vi "Execute Network Operation.vi"(7 "Operation":T1, 8 "error in (no error)":errorcluster, 10 "Message":string, 11 "Listener In.lvclass":refnum<class "Listener.lvclass">) -> (0 "error out":errorcluster, 3 "Listener Out.lvclass":refnum<class "Listener.lvclass">)   [LabVIEW 2019, in "Listener.lvclass"]
doc: "Reads/Writes data using the specified protocol.\nInput: \nListener Object\nMessage: The \"packet\" which will be sent through the selected protocol\nOpeartion: Read/Write operation on the specified protocol"
uses:
  Listener.lvclass
  ListenerClassControls/Operation.ctl
  Constants.vi
  <vilib>/Utility/error.llb/Error Cluster From Error Code.vi
  Protocols.lvlib
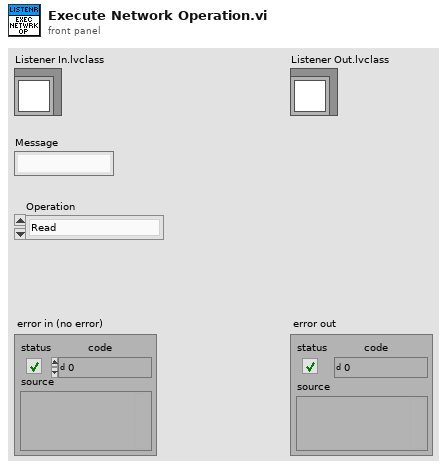
[diagram p1: front panel]
types:
  T1 = typedef "Listener.lvclass/Operation.ctl" = enum16{"Read", "Write"}
  T2 = enum16{"Standard", "Buffered", "CRLF", "Immediate"}
  T3 = typedef "Listener.lvclass/Protocol.ctl" = enum16{"RS-XXX", "AK RS-XXX", "VISA", "TCPIP", "AK TCPIP", "UDP", "GPIB ConvBox"}
  T4 = typedef "Listener.lvclass/UDP Data Structure.ctl" = cluster{"UDP connection ID":refnum<k16>, "Local Address":string, "Local Port":u16, "Target IP Address":string, "Target Port":u16, "Data":string}
  T5 = typedef "Listener.lvclass/TCP Data Structure.ctl" = cluster{"TCP|IP connection ID":refnum<k5>, "IP Address":string, "Port":u16, "Data":string}
  T6 = typedef "Listener.lvclass/AK TCP Data Structure.ctl" = cluster{"TCP|IP connection ID":refnum<k5>, "IP Address":string, "Port":u16, "Data":string, "Current Command Code":string}
  T7 = typedef "Listener.lvclass/VISA Data Structure.ctl" = cluster{"Protocol Ref Out":refnum<visa-resource-name>, "Listener Ref Out":refnum<visa-resource-name>, "Data Length":u32, "Data":string}
  T8 = typedef "Listener.lvclass/RS-xxx Data Structure.ctl" = cluster{"Protocol Port Ref":refnum<visa-resource-name>, "Listener Port Ref":refnum<visa-resource-name>, "Virtual COM Port Settings 1":cluster{"Port":string, "Baud Rate":u32, "Data Bits":u16, "Parity":enum16{"None", "Odd", "Even", "Mark", "Space"}, "Stop Bits":u16, "Flow Control":u16, "XON":enum16{"NUL", "SOH", "STX", "ETX", "EOT", "ENQ", "ACK", "BEL", "BS", "HT", "LF", "VT", "FF", "CR", "SO", "SI", "DLE", "DC1", "DC2", "DC3", "DC4", "NAK", "SYN", "ETB", "CAN", "EM", "SUB", "ESC", "FS", "GS", "RS", "US", "SP", "!", "\"", "#", "$", "%", "&", "'", "(", ")", "*", "+", ",", "- (-)", ".", "/", "0", "1", "2", "3", "4", "5", "6", "7", "8", "9", ":", ";", "<", "=", ">", "?", "@", "A", "B", "C", "D", "E", "F", "G", "H", "I", "J", "K", "L", "M", "N", "O", "P", "Q", "R", "S", "T", "U", "V", "W", "X", "Y", "Z", "[", "\\", "]", "^", "_", "`", "a", "b", "c", "d", "e", "f", "g", "h", "i", "j", "k", "l", "m", "n", "o", "p", "q", "r", "s", "t", "u", "v", "w", "x", "y", "z", "{", "|", "}", "~"}, "XOFF":enum16{"NUL", "SOH", "STX", "ETX", "EOT", "ENQ", "ACK", "BEL", "BS", "HT", "LF", "VT", "FF", "CR", "SO", "SI", "DLE", "DC1", "DC2", "DC3", "DC4", "NAK", "SYN", "ETB", "CAN", "EM", "SUB", "ESC", "FS", "GS", "RS", "US", "SP", "!", "\"", "#", "$", "%", "&", "'", "(", ")", "*", "+", ",", "- (-)", ".", "/", "0", "1", "2", "3", "4", "5", "6", "7", "8", "9", ":", ";", "<", "=", ">", "?", "@", "A", "B", "C", "D", "E", "F", "G", "H", "I", "J", "K", "L", "M", "N", "O", "P", "Q", "R", "S", "T", "U", "V", "W", "X", "Y", "Z", "[", "\\", "]", "^", "_", "`", "a", "b", "c", "d", "e", "f", "g", "h", "i", "j", "k", "l", "m", "n", "o", "p", "q", "r", "s", "t", "u", "v", "w", "x", "y", "z", "{", "|", "}", "~"}, "End Read on Termination Character":bool, "End Write on Termination Character":bool, "Termination Character":u8}, "Virtual COM Port Settings 2":cluster{"Port":string, "Baud Rate":u32, "Data Bits":u16, "Parity":enum16{"None", "Odd", "Even", "Mark", "Space"}, "Stop Bits":u16, "Flow Control":u16, "XON":enum16{"NUL", "SOH", "STX", "ETX", "EOT", "ENQ", "ACK", "BEL", "BS", "HT", "LF", "VT", "FF", "CR", "SO", "SI", "DLE", "DC1", "DC2", "DC3", "DC4", "NAK", "SYN", "ETB", "CAN", "EM", "SUB", "ESC", "FS", "GS", "RS", "US", "SP", "!", "\"", "#", "$", "%", "&", "'", "(", ")", "*", "+", ",", "- (-)", ".", "/", "0", "1", "2", "3", "4", "5", "6", "7", "8", "9", ":", ";", "<", "=", ">", "?", "@", "A", "B", "C", "D", "E", "F", "G", "H", "I", "J", "K", "L", "M", "N", "O", "P", "Q", "R", "S", "T", "U", "V", "W", "X", "Y", "Z", "[", "\\", "]", "^", "_", "`", "a", "b", "c", "d", "e", "f", "g", "h", "i", "j", "k", "l", "m", "n", "o", "p", "q", "r", "s", "t", "u", "v", "w", "x", "y", "z", "{", "|", "}", "~"}, "XOFF":enum16{"NUL", "SOH", "STX", "ETX", "EOT", "ENQ", "ACK", "BEL", "BS", "HT", "LF", "VT", "FF", "CR", "SO", "SI", "DLE", "DC1", "DC2", "DC3", "DC4", "NAK", "SYN", "ETB", "CAN", "EM", "SUB", "ESC", "FS", "GS", "RS", "US", "SP", "!", "\"", "#", "$", "%", "&", "'", "(", ")", "*", "+", ",", "- (-)", ".", "/", "0", "1", "2", "3", "4", "5", "6", "7", "8", "9", ":", ";", "<", "=", ">", "?", "@", "A", "B", "C", "D", "E", "F", "G", "H", "I", "J", "K", "L", "M", "N", "O", "P", "Q", "R", "S", "T", "U", "V", "W", "X", "Y", "Z", "[", "\\", "]", "^", "_", "`", "a", "b", "c", "d", "e", "f", "g", "h", "i", "j", "k", "l", "m", "n", "o", "p", "q", "r", "s", "t", "u", "v", "w", "x", "y", "z", "{", "|", "}", "~"}, "End Read on Termination Character":bool, "End Write on Termination Character":bool, "Termination Character":u8}, "Data":string, "Data Length":u32}
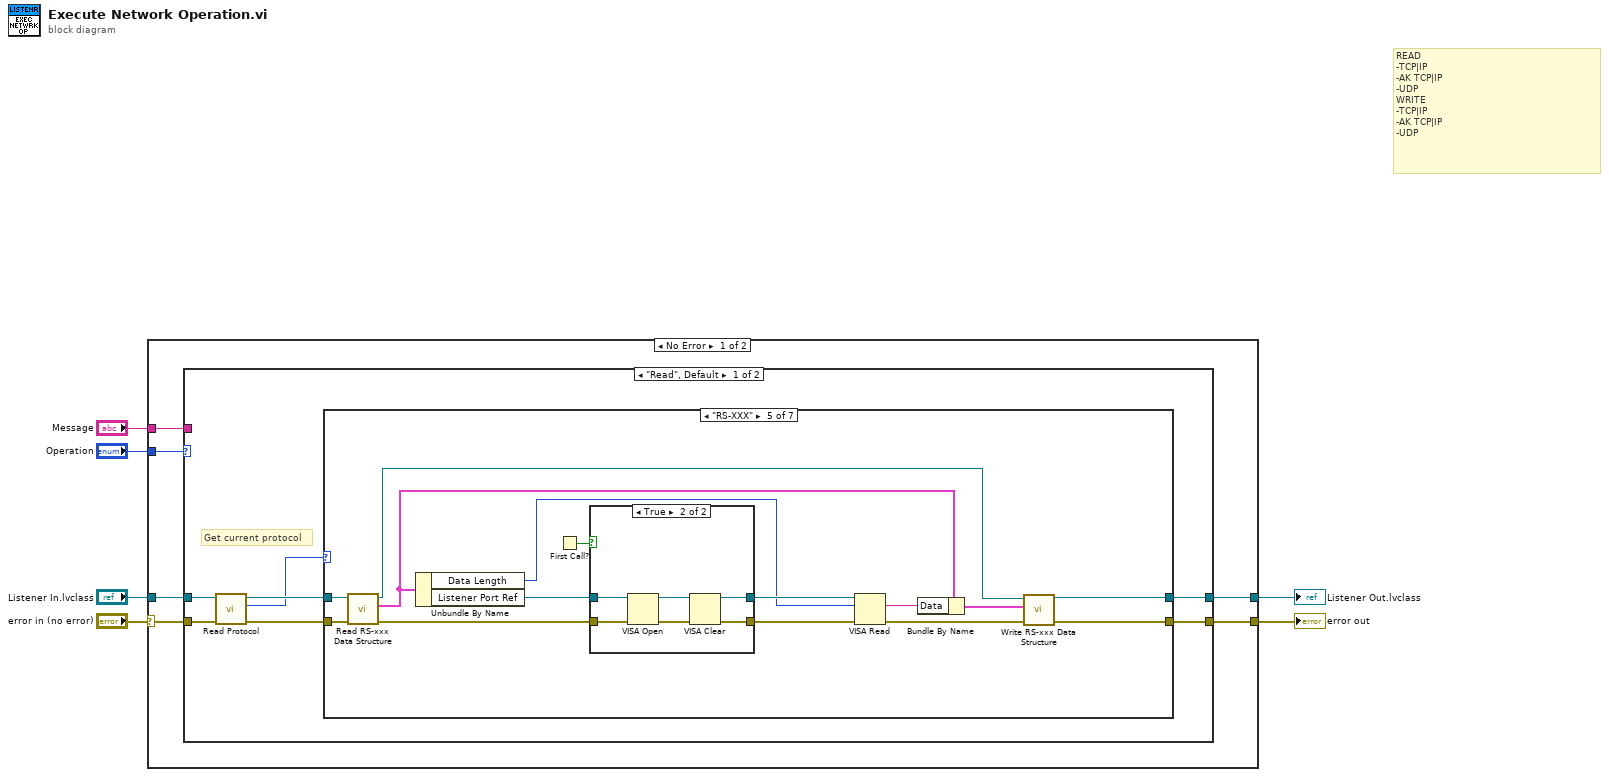
[diagram p0: block diagram]
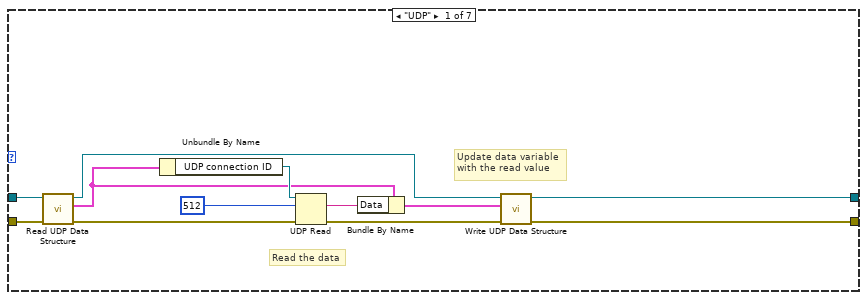
[diagram p2: hidden frame]
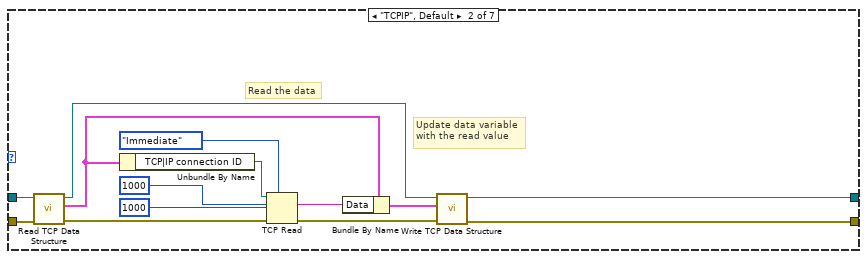
[diagram p3: hidden frame]
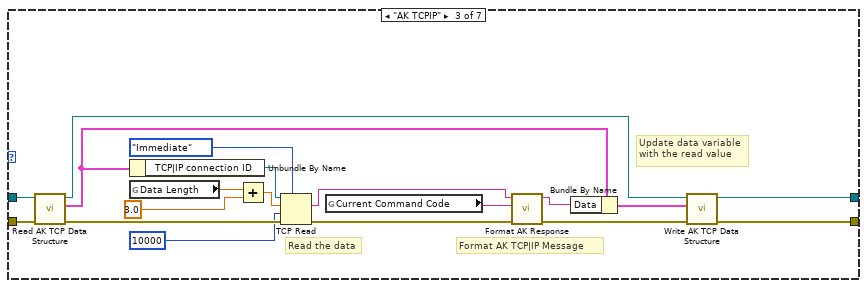
[diagram p4: hidden frame]
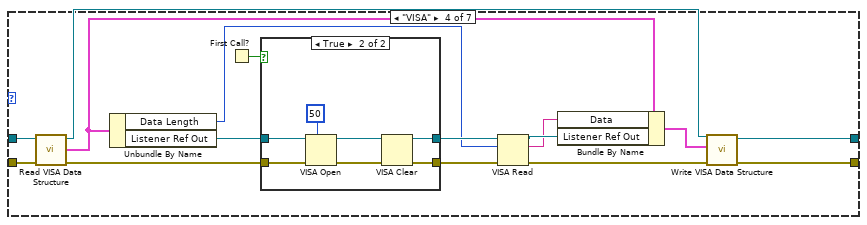
[diagram p5: hidden frame]
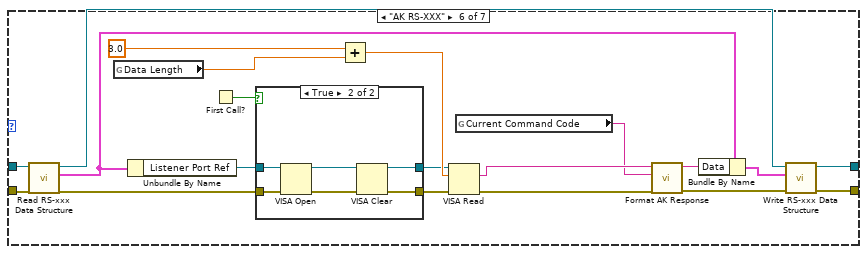
[diagram p8: hidden frame]
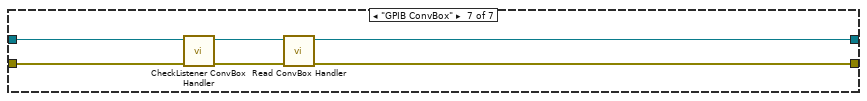
[diagram p10: hidden frame]
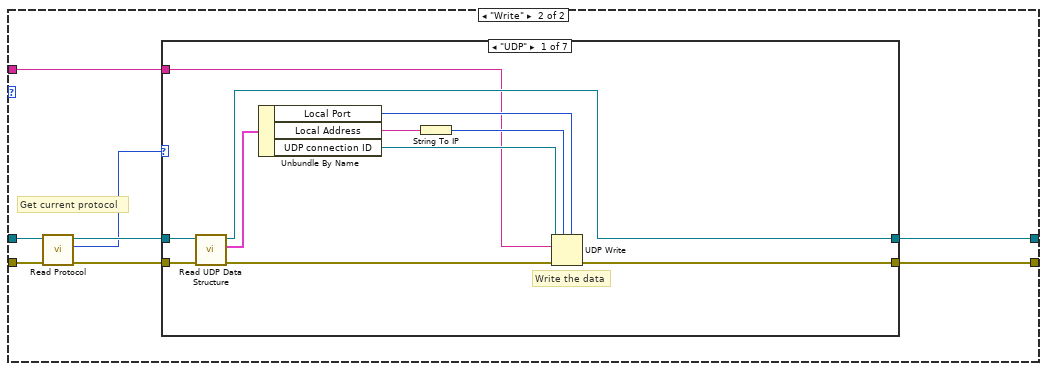
[diagram p11: hidden frame]
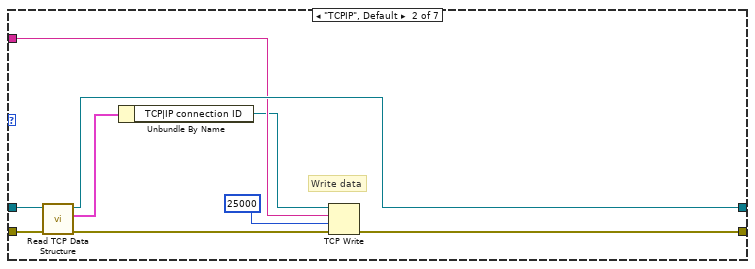
[diagram p12: hidden frame]
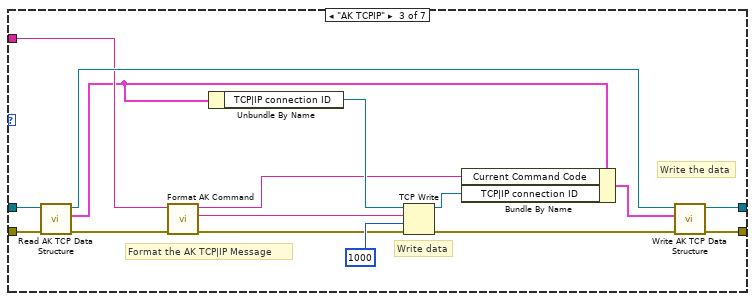
[diagram p13: hidden frame]
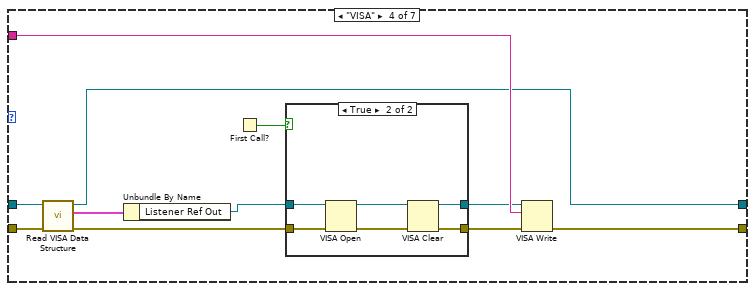
[diagram p14: hidden frame]
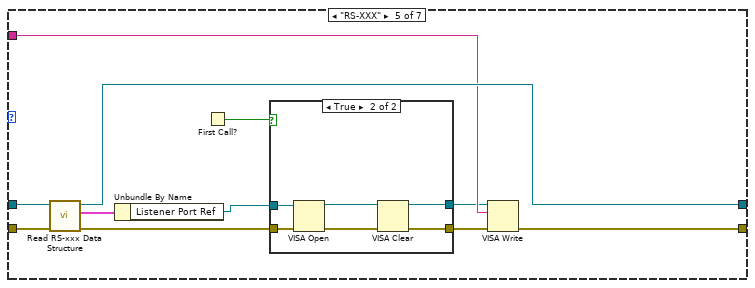
[diagram p16: hidden frame]
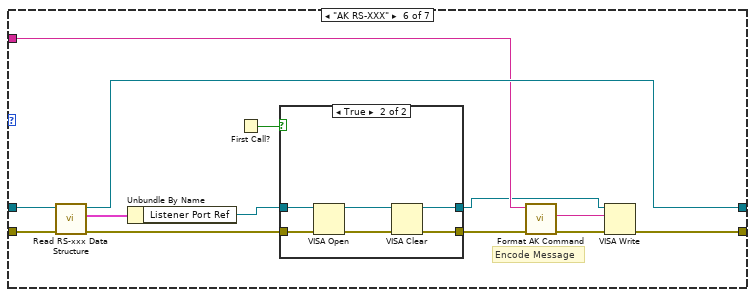
[diagram p18: hidden frame]
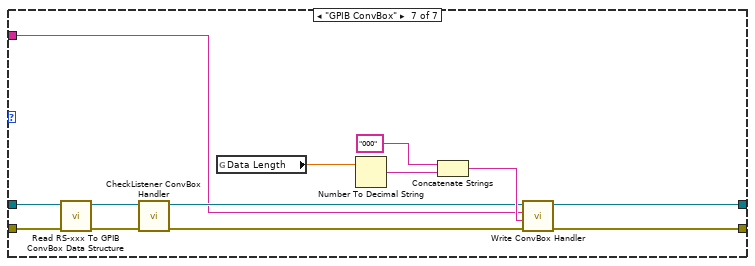
[diagram p20: hidden frame]
diagram:
  # "READ\n-TCP|IP\n-AK TCP|IP\n-UDP\nWRITE\n-TCP|IP\n-AK TCP|IP\n-UDP"
  n1 = case shown="No Error" "error in (no error)" {
    selector: "error in (no error)" -> [w9 w263]
    tunnel: "Listener In.lvclass" -> [w12 w264]
    tunnel: [w11 w263] -> w5
    tunnel: [w10 w264] -> w4
    tunnel: "Operation" -> [w8 _]
    tunnel: "Message" -> [w7 _]
    frame No Error {
      n2 = case shown="\"Read\", Default" w8 {
        tunnel: w9 -> [w19 w152]
        tunnel: w12 -> [w18 w149]
        tunnel: [w15 w153] -> w11
        tunnel: [w14 w154] -> w10
        tunnel: w7 -> [_ w147]
        frame "Read", Default {
          # "Get current protocol"
          n3 = call-dynamic "Read Protocol.vi"("error in (no error)"=w19, "Listener in"=w18) -> ("error out"=w17:errorcluster, "Protocol"=w13:T3, "Listener out"=w16:refnum<class "Listener.lvclass">)  [unwired: 7 in]
          n4 = case shown="\"RS-XXX\"" w13 {
            tunnel: w17 -> [w31 w45 w52 w79 w103 w130 w142]
            tunnel: w16 -> [w30 w44 w53 w80 w104 w129 w144]
            tunnel: [w28 w42 w50 w74 w97 w128 w145] -> w14
            tunnel: [w29 w43 w51 w77 w96 w113 w146] -> w15
            frame "UDP" {
              # "Read the data"
              # "Update data variable\nwith the read value"
              n5 = call-dynamic "Read UDP Data Structure.vi"("error in (no error)"=w31, "Listener in"=w30) -> ("error out"=w27:errorcluster, "UDP Data Structure"=w24:T4, "Listener out"=w21:refnum<class "Listener.lvclass">)  [unwired: 7 in]
              n6 = Unbundle By Name(w24) -> ("UDP connection ID"=w25:refnum<k16>)
              n7 = UDP Read(connection ID=w25, max size (548)=512, 8:w27) -> (data out=w23:string, error out=w22:errorcluster)  [unwired: 1 in, 3 out]
              n8 = Bundle By Name(cluster=w24, "Data"=w23) -> (w20:T4)
              n9 = call-dynamic "Write UDP Data Structure.vi"("error in (no error)"=w22, "UDP Data Structure"=w20, "Listener in"=w21) -> ("error out"=w29:errorcluster, "Listener out"=w28:refnum<class "Listener.lvclass">)  [unwired: 7 in]
            }
            frame "TCPIP", Default {
              # "Update data variable\nwith the read value"
              # "Read the data"
              n10 = call-dynamic "Read TCP Data Structure.vi"("error in (no error)"=w45, "Listener in"=w44) -> ("error out"=w40:errorcluster, "TCP|IP Data Structure"=w39:T5, "Listener out"=w35:refnum<class "Listener.lvclass">)  [unwired: 7 in]
              n11 = Unbundle By Name(w39) -> ("TCP|IP connection ID"=w34:refnum<k5>)
              n12 = TCP Read(connection ID=w34, bytes to read=1000, error in (no error)=w40, 7:T2."Immediate" ("mode (standard)"), 9:1000 ("timeout ms (25000)")) -> (data out=w38:string, error out=w36:errorcluster)  [unwired: 1 out]
              n13 = Bundle By Name(cluster=w39, "Data"=w38) -> (w37:T5)
              n14 = call-dynamic "Write TCP Data Structure.vi"("error in (no error)"=w36, "TCP|IP Data Structure"=w37, "Listener in"=w35) -> ("error out"=w43:errorcluster, "Listener out"=w42:refnum<class "Listener.lvclass">)  [unwired: 7 in]
            }
            frame "AK TCPIP" {
              # "Format AK TCP|IP Message"
              # "Update data variable\nwith the read value"
              # "Read the data"
              n15 = call-dynamic "Read AK TCP Data Structure.vi"("error in (no error)"=w52, "Listener in"=w53) -> ("error out"=w63:errorcluster, "TCP|IP Data Structure"=w60:T6, "Listener out"=w56:refnum<class "Listener.lvclass">)  [unwired: 7 in]
              n16 = Unbundle By Name(w60) -> ("TCP|IP connection ID"=w64:refnum<k5>)
              n17 = global read "Constants.vi" "Data Length"() -> (w49:dbl)
              n18 = Add(x=w49, y=3.0) -> (x+y=w47:dbl)
              n19 = TCP Read(connection ID=w64, bytes to read=w47, error in (no error)=w63, 7:T2."Immediate" ("mode (standard)"), 9:10000 ("timeout ms (25000)")) -> (data out=w61:string, error out=w62:errorcluster)  [unwired: 1 out]
              n20 = global read "Constants.vi" "Current Command Code"() -> (w46:string)
              n21 = call "Format AK Response.vi"("error in (no error)"=w62, "Current Command Code"=w46, "Response"=w61) -> ("error out"=w58:errorcluster, "Data"=w59:string)  [unwired: 7 in]
              n22 = Bundle By Name(cluster=w60, "Data"=w59) -> (w57:T6)
              n23 = call-dynamic "Write AK TCP Data Structure.vi"("error in (no error)"=w58, "TCP|IP Data Structure"=w57, "Listener in"=w56) -> ("error out"=w51:errorcluster, "Listener out"=w50:refnum<class "Listener.lvclass">)  [unwired: 7 in]
            }
            frame "VISA" {
              n24 = call-dynamic "Read VISA Data Structure.vi"("error in (no error)"=w79, "Listener in"=w80) -> ("error out"=w71:errorcluster, "VISA Data Structure"=w78:T7, "Listener out"=w75:refnum<class "Listener.lvclass">)  [unwired: 7 in]
              n25 = Unbundle By Name(w78) -> ("Data Length"=w68:u32, "Listener Ref Out"=w67:refnum<visa-resource-name>)
              n26 = First Call?() -> (First Call?: T/F=w72:bool)
              n27 = case shown="True" w72 {
                tunnel: w67 -> [w82 w89]
                tunnel: w71 -> [w81 w88]
                tunnel: [w81 w87] -> w70
                tunnel: [w82 w86] -> w69
                frame False {
                }
                frame True {
                  n28 = VISA Open(timeout (0)=u32 50 ("VISA Open timeout (0)"), error in (no error)=w88, VISA resource name=w89) -> (VISA resource name=w84:refnum<visa-resource-name>, error out=w85:errorcluster)  [unwired: 2 in]
                  n29 = VISA Clear(VISA resource name=w84, error in (no error)=w85) -> (VISA resource name out=w86:refnum<visa-resource-name>, error out=w87:errorcluster)
                }
              }
              n30 = VISA Read(VISA resource name=w69, byte count=w68, error in (no error)=w70) -> (VISA resource name out=w66:refnum<visa-resource-name>, read buffer=w65:string, error out=w73:errorcluster)  [unwired: 1 out]
              n31 = Bundle By Name(cluster=w78, "Data"=w65, "Listener Ref Out"=w66) -> (w76:T7)
              n32 = call-dynamic "Write VISA Data Structure.vi"("error in (no error)"=w73, "VISA Data Structure"=w76, "Listener in"=w75) -> ("error out"=w77:errorcluster, "Listener out"=w74:refnum<class "Listener.lvclass">)  [unwired: 7 in]
            }
            frame "RS-XXX" {
              n33 = call-dynamic "Read RS-xxx Data Structure.vi"("error in (no error)"=w103, "Listener in"=w104) -> ("error out"=w93:errorcluster, "RS-xxx Data Structure"=w102:T8, "Listener out"=w99:refnum<class "Listener.lvclass">)  [unwired: 7 in]
              n34 = Unbundle By Name(w102) -> ("Data Length"=w90:u32, "Listener Port Ref"=w94:refnum<visa-resource-name>)
              n35 = First Call?() -> (First Call?: T/F=w95:bool)
              n36 = case shown="True" w95 {
                tunnel: w94 -> [w106 w112]
                tunnel: w93 -> [w105 w110]
                tunnel: [w105 w108] -> w92
                tunnel: [w106 w107] -> w91
                frame False {
                }
                frame True {
                  n37 = VISA Open(error in (no error)=w110, VISA resource name=w112) -> (VISA resource name=w111:refnum<visa-resource-name>, error out=w109:errorcluster)  [unwired: 3 in]
                  n38 = VISA Clear(VISA resource name=w111, error in (no error)=w109) -> (VISA resource name out=w107:refnum<visa-resource-name>, error out=w108:errorcluster)
                }
              }
              n39 = VISA Read(VISA resource name=w91, byte count=w90, error in (no error)=w92) -> (read buffer=w101:string, error out=w98:errorcluster)  [unwired: 2 out]
              n40 = Bundle By Name(cluster=w102, "Data"=w101) -> (w100:T8)
              n41 = call-dynamic "Write RS-xxx Data Structure.vi"("error in (no error)"=w98, "RS-xxx Data Structure"=w100, "Listener in"=w99) -> ("error out"=w96:errorcluster, "Listener out"=w97:refnum<class "Listener.lvclass">)  [unwired: 7 in]
            }
            frame "AK RS-XXX" {
              n42 = call-dynamic "Read RS-xxx Data Structure.vi"("error in (no error)"=w130, "Listener in"=w129) -> ("error out"=w117:errorcluster, "RS-xxx Data Structure"=w131:T8, "Listener out"=w132:refnum<class "Listener.lvclass">)  [unwired: 7 in]
              n43 = global read "Constants.vi" "Data Length"() -> (w124:dbl)
              n44 = Unbundle By Name(w131) -> ("Listener Port Ref"=w116:refnum<visa-resource-name>)
              n45 = First Call?() -> (First Call?: T/F=w118:bool)
              n46 = case shown="True" w118 {
                tunnel: w116 -> [w134 w140]
                tunnel: w117 -> [w133 w139]
                tunnel: [w133 w137] -> w114
                tunnel: [w134 w136] -> w115
                frame False {
                }
                frame True {
                  n47 = VISA Open(error in (no error)=w139, VISA resource name=w140) -> (VISA resource name=w135:refnum<visa-resource-name>, error out=w138:errorcluster)  [unwired: 3 in]
                  n48 = VISA Clear(VISA resource name=w135, error in (no error)=w138) -> (VISA resource name out=w136:refnum<visa-resource-name>, error out=w137:errorcluster)
                }
              }
              n49 = Add(x=3.0 ("y"), y=w124) -> (x+y=w125:dbl)
              n50 = VISA Read(VISA resource name=w115, byte count=w125, error in (no error)=w114) -> (read buffer=w122:string, error out=w120:errorcluster)  [unwired: 2 out]
              n51 = global read "Constants.vi" "Current Command Code"() -> (w121:string)
              n52 = call "Format AK Response.vi"("error in (no error)"=w120, "Current Command Code"=w121, "Response"=w122) -> ("error out"=w119:errorcluster, "Data"=w127:string)  [unwired: 7 in]
              n53 = Bundle By Name(cluster=w131, "Data"=w127) -> (w126:T8)
              n54 = call-dynamic "Write RS-xxx Data Structure.vi"("error in (no error)"=w119, "RS-xxx Data Structure"=w126, "Listener in"=w132) -> ("error out"=w113:errorcluster, "Listener out"=w128:refnum<class "Listener.lvclass">)  [unwired: 7 in]
            }
            frame "GPIB ConvBox" {
              n55 = call "CheckListener ConvBox Handler.vi"("error in (no error)"=w142, "Listener in"=w144) -> ("error out"=w141:errorcluster, "Listener out"=w143:refnum<class "Listener.lvclass">)  [unwired: 8 in]
              n56 = call "Read ConvBox Handler.vi"("error in (no error)"=w141, "Listener in"=w143) -> ("error out"=w146:errorcluster, "Listener out"=w145:refnum<class "Listener.lvclass">)  [unwired: 8 in]
            }
          }
        }
        frame "Write" {
          # "Get current protocol"
          n57 = call-dynamic "Read Protocol.vi"("error in (no error)"=w152, "Listener in"=w149) -> ("error out"=w151:errorcluster, "Protocol"=w148:T3, "Listener out"=w150:refnum<class "Listener.lvclass">)  [unwired: 7 in]
          n58 = case shown="\"UDP\"" w148 {
            tunnel: [w162 w174 w178 w197 w216 w238 w262] -> w154
            tunnel: [w163 w173 w177 w196 w219 w239 w261] -> w153
            tunnel: w150 -> [w164 w171 w176 w201 w217 w241 w255]
            tunnel: w151 -> [w165 w172 w179 w200 w218 w240 w254]
            tunnel: w147 -> [w155 w170 w180 w199 w215 w235 w250]
            frame "UDP" {
              # "Write the data"
              n59 = call-dynamic "Read UDP Data Structure.vi"("error in (no error)"=w165, "Listener in"=w164) -> ("error out"=w159:errorcluster, "UDP Data Structure"=w161:T4, "Listener out"=w162:refnum<class "Listener.lvclass">)  [unwired: 7 in]
              n60 = Unbundle By Name(w161) -> ("Local Port"=w158:u16, "Local Address"=w157:string, "UDP connection ID"=w160:refnum<k16>)
              n61 = String To IP(1:w157) -> (0:w156:u32)
              n62 = UDP Write(address=w156, port or service name=w158, connection ID=w160, data in=w155, 8:w159) -> (error out=w163:errorcluster)  [unwired: 1 in, 1 out]
            }
            frame "TCPIP", Default {
              # "Write data"
              n63 = call-dynamic "Read TCP Data Structure.vi"("error in (no error)"=w172, "Listener in"=w171) -> ("error out"=w166:errorcluster, "TCP|IP Data Structure"=w168:T5, "Listener out"=w174:refnum<class "Listener.lvclass">)  [unwired: 7 in]
              n64 = Unbundle By Name(w168) -> ("TCP|IP connection ID"=w169:refnum<k5>)
              n65 = TCP Write(connection ID=w169, data in=w170, error in (no error)=w166, 9:25000 ("timeout ms (25000)")) -> (error out=w173:errorcluster)  [unwired: 2 out]
            }
            frame "AK TCPIP" {
              # "Format the AK TCP|IP Message"
              # "Write the data"
              # "Write data"
              n66 = call-dynamic "Read AK TCP Data Structure.vi"("error in (no error)"=w179, "Listener in"=w176) -> ("error out"=w187:errorcluster, "TCP|IP Data Structure"=w175:T6, "Listener out"=w186:refnum<class "Listener.lvclass">)  [unwired: 7 in]
              n67 = call "Format AK Command.vi"("error in (no error)"=w187, "String in"=w180) -> ("error out"=w188:errorcluster, "Command"=w184:string, "Command Code"=w183:string)  [unwired: 7 in]
              n68 = Unbundle By Name(w175) -> ("TCP|IP connection ID"=w190:refnum<k5>)
              n69 = TCP Write(connection ID=w190, data in=w184, error in (no error)=w188, 9:1000 ("timeout ms (25000)")) -> (connection ID out=w182:refnum<k5>, error out=w185:errorcluster)  [unwired: 1 out]
              n70 = Bundle By Name(cluster=w175, "Current Command Code"=w183, "TCP|IP connection ID"=w182) -> (w181:T6)
              n71 = call-dynamic "Write AK TCP Data Structure.vi"("error in (no error)"=w185, "TCP|IP Data Structure"=w181, "Listener in"=w186) -> ("error out"=w177:errorcluster, "Listener out"=w178:refnum<class "Listener.lvclass">)  [unwired: 7 in]
            }
            frame "VISA" {
              n72 = call-dynamic "Read VISA Data Structure.vi"("error in (no error)"=w200, "Listener in"=w201) -> ("error out"=w194:errorcluster, "VISA Data Structure"=w198:T7, "Listener out"=w197:refnum<class "Listener.lvclass">)  [unwired: 7 in]
              n73 = Unbundle By Name(w198) -> ("Listener Ref Out"=w191:refnum<visa-resource-name>)
              n74 = First Call?() -> (First Call?: T/F=w195:bool)
              n75 = case shown="True" w195 {
                tunnel: w191 -> [w203 w209]
                tunnel: w194 -> [w202 w208]
                tunnel: [w202 w207] -> w192
                tunnel: [w203 w206] -> w193
                frame False {
                }
                frame True {
                  n76 = VISA Open(error in (no error)=w208, VISA resource name=w209) -> (VISA resource name=w205:refnum<visa-resource-name>, error out=w204:errorcluster)  [unwired: 3 in]
                  n77 = VISA Clear(VISA resource name=w205, error in (no error)=w204) -> (VISA resource name out=w206:refnum<visa-resource-name>, error out=w207:errorcluster)
                }
              }
              n78 = VISA Write(VISA resource name=w193, write buffer=w199, error in (no error)=w192) -> (error out=w196:errorcluster)  [unwired: 2 out]
            }
            frame "RS-XXX" {
              n79 = call-dynamic "Read RS-xxx Data Structure.vi"("error in (no error)"=w218, "Listener in"=w217) -> ("error out"=w211:errorcluster, "RS-xxx Data Structure"=w220:T8, "Listener out"=w216:refnum<class "Listener.lvclass">)  [unwired: 7 in]
              n80 = Unbundle By Name(w220) -> ("Listener Port Ref"=w213:refnum<visa-resource-name>)
              n81 = First Call?() -> (First Call?: T/F=w214:bool)
              n82 = case shown="True" w214 {
                tunnel: w211 -> [w222 w228]
                tunnel: [w222 w226] -> w210
                tunnel: [w221 w225] -> w212
                tunnel: w213 -> [w221 w223]
                frame False {
                }
                frame True {
                  n83 = VISA Open(error in (no error)=w228, VISA resource name=w223) -> (VISA resource name=w224:refnum<visa-resource-name>, error out=w227:errorcluster)  [unwired: 3 in]
                  n84 = VISA Clear(VISA resource name=w224, error in (no error)=w227) -> (VISA resource name out=w225:refnum<visa-resource-name>, error out=w226:errorcluster)
                }
              }
              n85 = VISA Write(VISA resource name=w212, write buffer=w215, error in (no error)=w210) -> (error out=w219:errorcluster)  [unwired: 2 out]
            }
            frame "AK RS-XXX" {
              # "Encode Message"
              n86 = call-dynamic "Read RS-xxx Data Structure.vi"("error in (no error)"=w240, "Listener in"=w241) -> ("error out"=w232:errorcluster, "RS-xxx Data Structure"=w236:T8, "Listener out"=w238:refnum<class "Listener.lvclass">)  [unwired: 7 in]
              n87 = Unbundle By Name(w236) -> ("Listener Port Ref"=w231:refnum<visa-resource-name>)
              n88 = First Call?() -> (First Call?: T/F=w233:bool)
              n89 = case shown="True" w233 {
                tunnel: w232 -> [w243 w249]
                tunnel: [w243 w247] -> w230
                tunnel: [w242 w246] -> w229
                tunnel: w231 -> [w242 w244]
                frame False {
                }
                frame True {
                  n90 = VISA Open(error in (no error)=w249, VISA resource name=w244) -> (VISA resource name=w245:refnum<visa-resource-name>, error out=w248:errorcluster)  [unwired: 3 in]
                  n91 = VISA Clear(VISA resource name=w245, error in (no error)=w248) -> (VISA resource name out=w246:refnum<visa-resource-name>, error out=w247:errorcluster)
                }
              }
              n92 = call "Format AK Command.vi"("error in (no error)"=w230, "String in"=w235) -> ("error out"=w234:errorcluster, "Command"=w237:string)  [unwired: 7 in, 1 out]
              n93 = VISA Write(VISA resource name=w229, write buffer=w237, error in (no error)=w234) -> (error out=w239:errorcluster)  [unwired: 2 out]
            }
            frame "GPIB ConvBox" {
              n94 = call-dynamic "Read RS-xxx To GPIB ConvBox Data Structure.vi"("error in (no error)"=w254, "Listener in"=w255) -> ("error out"=w253:errorcluster, "Listener out"=w252:refnum<class "Listener.lvclass">)  [unwired: 7 in, 1 out]
              n95 = call "CheckListener ConvBox Handler.vi"("error in (no error)"=w253, "Listener in"=w252) -> ("error out"=w251:errorcluster, "Listener out"=w256:refnum<class "Listener.lvclass">)  [unwired: 8 in]
              n96 = global read "Constants.vi" "Data Length"() -> (w260:dbl)
              n97 = Number To Decimal String(number=w260) -> (decimal integer string=w259:string)  [unwired: 1 in]
              n98 = Concatenate Strings("000" ("string"), w259) -> (w257:string)
              n99 = call "Write ConvBox Handler.vi"("error in (no error)"=w251, "Data Length"=w257, "Data"=w250, "Listener in"=w256) -> ("error out"=w261:errorcluster, "Listener out"=w262:refnum<class "Listener.lvclass">)  [unwired: 6 in]
            }
          }
        }
      }
    }
    frame Error {
    }
  }
  "Listener Out.lvclass" <- w4
  "error out" <- w5
